vi "Read Config File.vi"(8 "error in (no error)":errorcluster) -> (0 "error out":errorcluster, 2 "ConfigFile":path, 3 "Data Value Reference out":T1)   [LabVIEW 2011]
uses:
  Controls/Options DVR.ctl
  Controls/Options.ctl
  <vilib>/Utility/config.llb/Read Key (Path).vi
  <vilib>/Utility/config.llb/Read Key (Boolean).vi
  <vilib>/Utility/config.llb/NI_LVConfig.lvlib
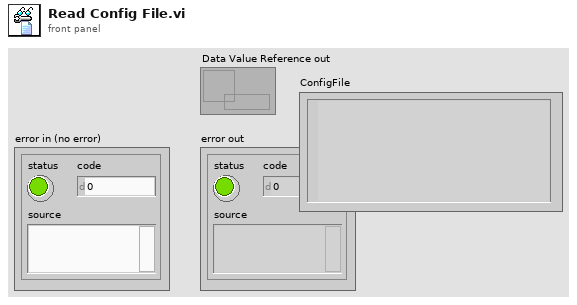
[diagram p1: front panel]
types:
  T1 = typedef "Options DVR.ctl" = refnum<data-value>
  T2 = typedef "Options.ctl" = cluster{"Logging?":bool, "TimeStamp?":bool, "LogInCSVDir?":bool, "LogDir":path}
  T3 = typedef "NI_LVConfig.lvlib/Config Data RefNum.ctl" = refnum<k1>
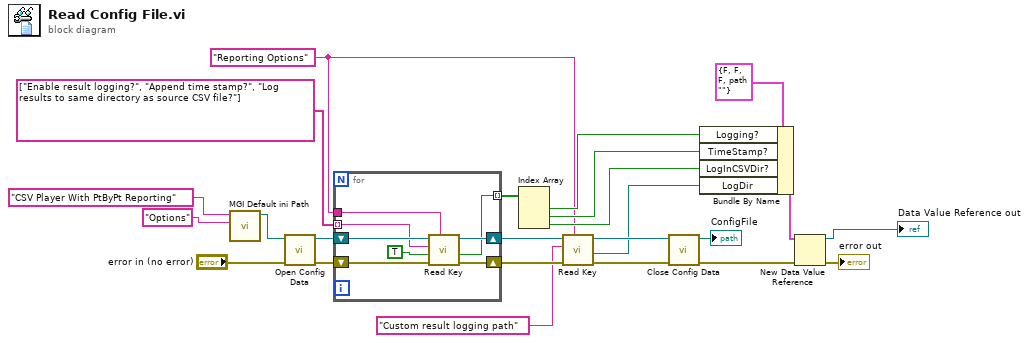
[diagram p0: block diagram]
diagram:
  w5 = "Reporting Options" ("section")
  n1 = call <userlib>:"MGI Default ini Path.vi"("File Name (Caller's Prefix)"="Options", "Folder Name (Caller's Prefix)"="CSV Player With PtByPt Reporting") -> ("Path"=w1:path)  [unwired: 9 in]
  n2 = call <vilib>:"Open Config Data.vi"("error in (no error)"="error in (no error)", "configuration file path"=w1) -> ("error out"=w22:errorcluster, "refnum"=w21:T3)  [unwired: 7 in, 1 out]
  n3 = for {
    shift-right: [w30] -> w19
    shift-left: w22 -> [w32]
    shift-right: [w29] -> w18
    shift-left: w21 -> [w31]
    tunnel: w5 -> [w28]
    tunnel: string[] ["Enable result logging?", "Append time stamp?", "Log results to same directory as source CSV file?"] -> [w27] mode=indexing
    tunnel: [w25] -> w10 mode=indexing
    n4 = call-poly <vilib>:"Read Key.vi"("section"=w28, "error in (no error)"=w32, "default value"=TRUE, "key"=w27, "refnum"=w31) -> ("error out"=w30:errorcluster, "value"=w25:bool, "refnum out"=w29:T3)  [unwired: 3 in, 1 out]
  }
  n5 = Index Array(array=w10) -> (element #1=w9:bool, element #2=w8:bool, element #3=w7:bool)  [unwired: 3 in]
  n6 = call-poly <vilib>:"Read Key.vi"("section"=w5, "error in (no error)"=w19, "key"="Custom result logging path" ("section"), "refnum"=w18) -> ("error out"=w16:errorcluster, "value"=w6:path, "refnum out"=w17:T3)  [unwired: 4 in, 1 out]
  n7 = call <vilib>:"Close Config Data.vi"("error in (no error)"=w16, "refnum"=w17) -> ("error out"=w15:errorcluster, "file path"=→"ConfigFile":path)  [unwired: 8 in]
  n8 = Bundle By Name(cluster=T2 {"Logging?"=FALSE, "TimeStamp?"=FALSE, "LogInCSVDir?"=FALSE, "LogDir"=path ""} ("Options"), "Logging?"=w9, "TimeStamp?"=w8, "LogInCSVDir?"=w7, "LogDir"=w6) -> (w12:T2)
  n9 = New Data Value Reference(data value=w12, error in=w15) -> (data value reference=→"Data Value Reference out":refnum<data-value>, error out=→"error out":errorcluster)
